vi "XIPIN_AXI_Performance_Monitor_5_0.vi"   [LabVIEW 2017]
doc: "AXI Performance Monitor\n------------------------------------\n<b>Need License</b> : No\n<b>Interface</b> : AXI4 AXI4-Stream"
uses:
  <vilib>/rvi/XilinxIP/XIPIN_XNode/niFpgaXIPIN.xnode
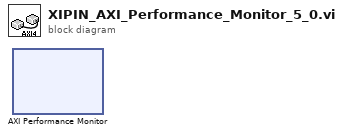
[diagram p0: block diagram]
diagram:
  n1 = xnode ("AXI Performance Monitor")() -> ()
